vi "Eagle_RT Globals.vi"() -> ()   [LabVIEW 2015]
panel:
  in  "AB Lookup":cluster{"x":dbl, "y":dbl}[](array[cluster])=[{"x"=1.0, "y"=1.0}, {"x"=2.0, "y"=2.0}, {"x"=3.0, "y"=3.0}, {"x"=4.0, "y"=4.0}, {"x"=5.0, "y"=5.0}]
  in  "RB Lookup":cluster{"x":dbl, "y":dbl}[](array[cluster])=[{"x"=1.0, "y"=1.0}, {"x"=2.0, "y"=2.0}, {"x"=3.0, "y"=3.0}, {"x"=4.0, "y"=4.0}, {"x"=5.0, "y"=5.0}]
  in  "LR Lookup":cluster{"x":dbl, "y":dbl}[](array[cluster])=[{"x"=1.0, "y"=1.0}, {"x"=2.0, "y"=2.0}, {"x"=3.0, "y"=3.0}, {"x"=4.0, "y"=4.0}, {"x"=5.0, "y"=5.0}]
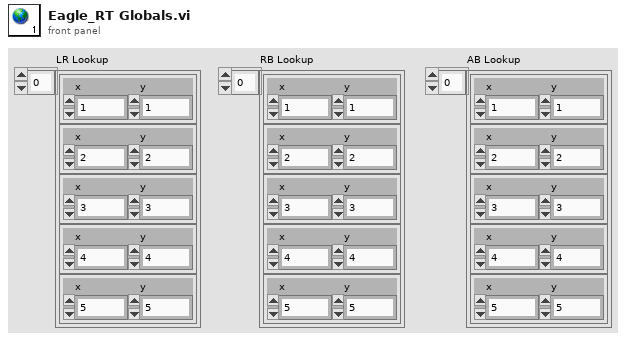
[diagram p1: front panel]
diagram:
